vi "getPositionWithTime_32Bit.vi"(0 "connection ID":refnum<k5>, 1 "axis":i32, 5 "error in":errorcluster) -> (14 "connection ID":refnum<k5>, 15 "axis_out":i32, 16 "Monotonic_time_sec":i32, 17 "Monotonic_time_nsec":i32, 18 "position":dbl, 19 "error out":errorcluster)   [LabVIEW 2016, in "AMC_VIs.lvlib"]
doc: "This function gets the current position of the positioner and provides time-information to the position."
uses:
  AMC_VIs.lvlib
panel:
  out "params_cluster":cluster{"axis":i32}
  in  "Params_cluster":cluster{"integer":i32}
  in  "results_cluster":T1
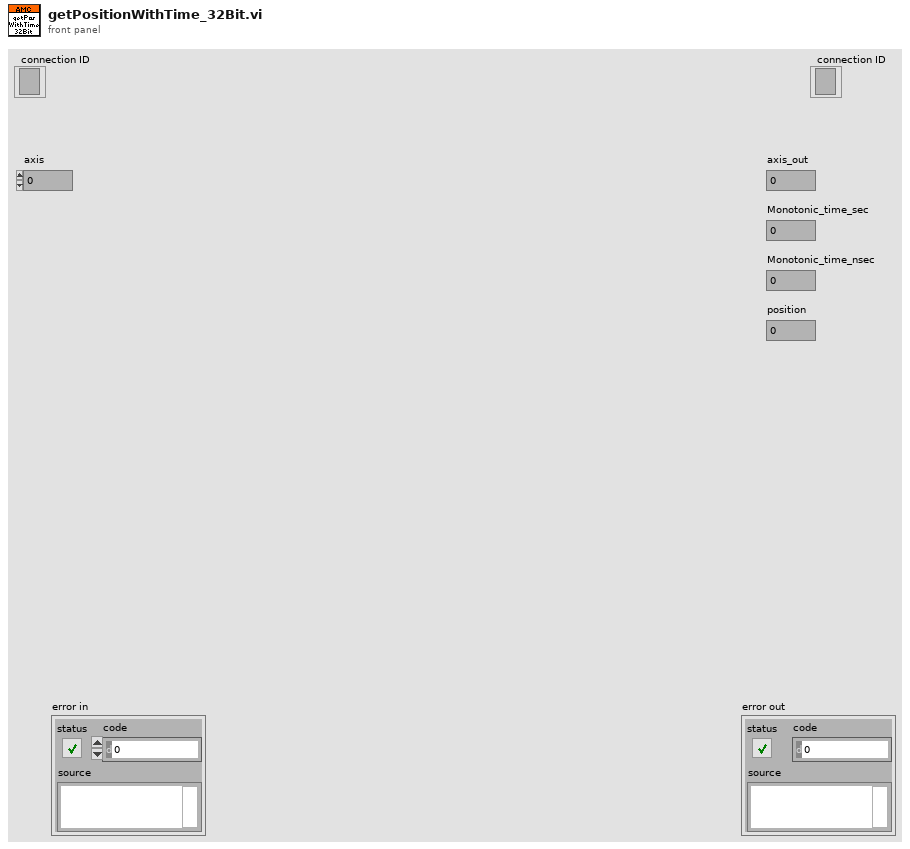
[diagram p1: front panel]
types:
  T1 = cluster{"errNo":i32, "Monotonic_time_sec":i32, "Monotonic_time_nsec":i32, "position":dbl}
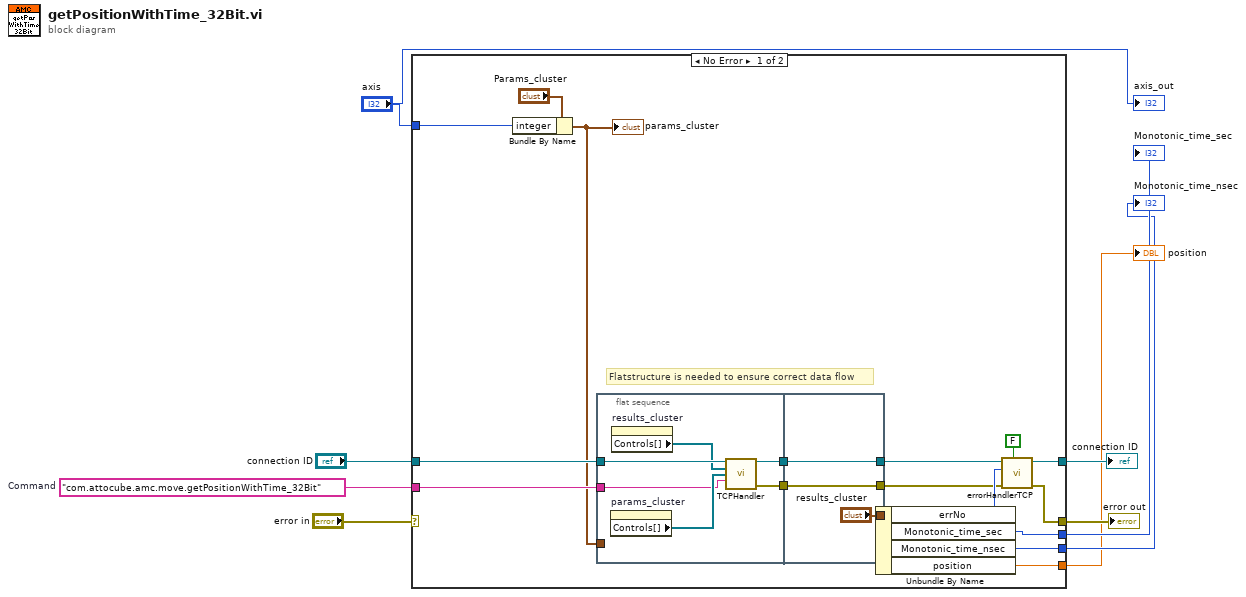
[diagram p0: block diagram]
diagram:
  w5 = "com.attocube.amc.move.getPositionWithTime_32Bit"  # Command
  n1 = case shown="No Error" "error in" {
    selector: "error in" -> [_ w37]
    tunnel: [w24 w37] -> w9
    tunnel: [w26 w36] -> w8
    tunnel: "connection ID" -> [w23 w36]
    tunnel: w5 -> [w17 _]
    tunnel: "axis" -> [w13 _]
    tunnel: [w12 _] -> w3
    tunnel: [w11 _] -> w2
    tunnel: [w10 _] -> w1
    frame No Error {
      # "Flatstructure is needed to ensure correct data flow"
      n2 = Bundle By Name(cluster="Params_cluster", "integer"=w13) -> (w14:cluster{"integer":i32})
      "params_cluster" <- w14
      n3 = flat-sequence {
        tunnel: [w31] -> w19
        tunnel: w23 -> [w32]
        tunnel: w17 -> [w28]
        tunnel: [w27] -> w15
        tunnel: w14 -> [_]
        tunnel: ["results_cluster"] -> w20
        tunnel: [w35] -> w22
        tunnel: w19 -> [w35]
        tunnel: [w33] -> w16
        tunnel: w15 -> [w33]
        frame #0 {
          n4 = property on="params_cluster" class="Clust (strict)"() -> ("Controls[]"=w29:refnum<vi>[])  [unwired: 2 in, 2 out]
          n5 = property on="results_cluster" class="Clust (strict)"() -> ("Controls[]"=w30:refnum<vi>[])  [unwired: 2 in, 2 out]
          n6 = call "TCPHandler.vi"("connection ID"=w32, "results_cluster"=w30, "params_cluster"=w29, "method"=w28) -> ("connection ID"=w31:refnum<k5>, "error"=w27:errorcluster)  [unwired: 8 in, 2 out]
        }
        frame #1 {
        }
      }
      n7 = Unbundle By Name(w20) -> ("errNo"=w21:i32, "Monotonic_time_sec"=w12:i32, "Monotonic_time_nsec"=w11:i32, "position"=w10:dbl)
      n8 = call "errorHandlerTCP.vi"("show popup"=FALSE, "error in"=w16, "error number"=w21, "connection ID"=w22) -> ("error out"=w24:errorcluster, "connection ID"=w26:refnum<k5>)  [unwired: 6 in]
    }
    frame Error {
    }
  }
  "error out" <- w9
  "connection ID" <- w8
  "Monotonic_time_sec" <- w3
  "Monotonic_time_nsec" <- w2
  "position" <- w1
  "axis_out" <- "axis"
